vi "qa_min_0@11.vi"(0 "Pu":dbl, 1 "T":dbl, 2 "Cc":dbl, 3 "Pénalité":dbl, 4 "Cpc":dbl, 5 "error in (no error)":errorcluster caption="err in") -> (14 "Qa min":dbl, 19 "error out":errorcluster caption="err out")   [LabVIEW 2010, in "lv_07.lvlib"]
doc: "Calcul de la qté minimum à consommer à l'année pour justifier du stockage de la pièce."
uses:
  lv_07.lvlib
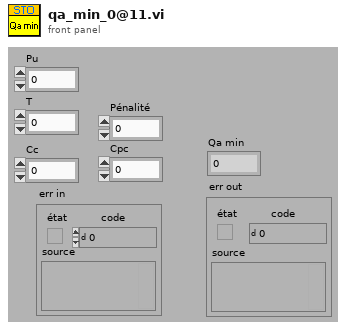
[diagram p1: front panel]
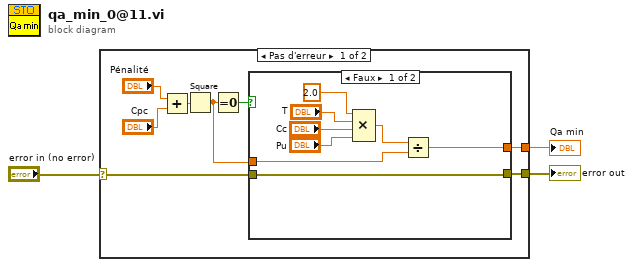
[diagram p0: block diagram]
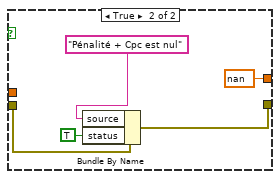
[diagram p2: hidden frame]
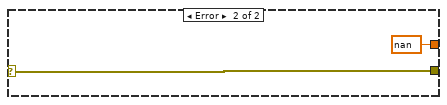
[diagram p3: hidden frame]
diagram:
  n1 = case shown="Pas d'erreur" "error in (no error)" {
    selector: "error in (no error)" -> [w8 w26]
    tunnel: [w7 w26] -> w2
    tunnel: [w4 nan] -> w1
    frame No Error {
      n2 = Add(x="Pénalité", y="Cpc") -> (x+y=w6:dbl)
      n3 = Square(x=w6) -> (x^2=w5:dbl)
      n4 = Equal To 0?(x=w5) -> (x = 0?=w9:bool)
      n5 = case shown="Faux" w9 {
        tunnel: w8 -> [w12 w24]
        tunnel: [w12 w21] -> w7
        tunnel: w5 -> [w14 _]
        tunnel: [w13 nan] -> w4
        frame False {
          n6 = Compound Arithmetic op=MULTIPLY(2.0, "T", "Cc", "Pu") -> (w16:dbl)
          n7 = Divide(x=w16, y=w14) -> (x/y=w13:dbl)
        }
        frame True {
          n8 = Bundle By Name(cluster=w24, "source"="Pénalité + Cpc est nul", "status"=TRUE) -> (w21:errorcluster)
        }
      }
    }
    frame Error {
    }
  }
  "error out" <- w2
  "Qa min" <- w1
